vi "Load Products.vi"(8 "error in (no error)":errorcluster, 11 "Spanish Picker in":refnum<class "Spanish Picker.lvclass">) -> (0 "error out":errorcluster, 3 "Spanish Picker out":refnum<class "Spanish Picker.lvclass">)   [LabVIEW 2020, in "Spanish Picker.lvlib" / "Spanish Picker.lvclass"]
uses:
  Spanish Picker.lvclass
  D:/Storage/Source Code/Clase AF/ClaseAF/05 AF Camera/Products Picker/Products Picker.lvclass
  Products Picker/Products Picker.lvclass/Products Picker.ctl
  Products Picker/Products Picker.lvclass
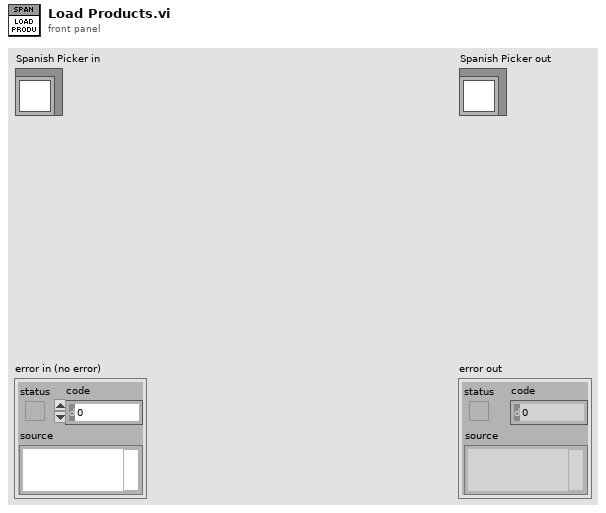
[diagram p1: front panel]
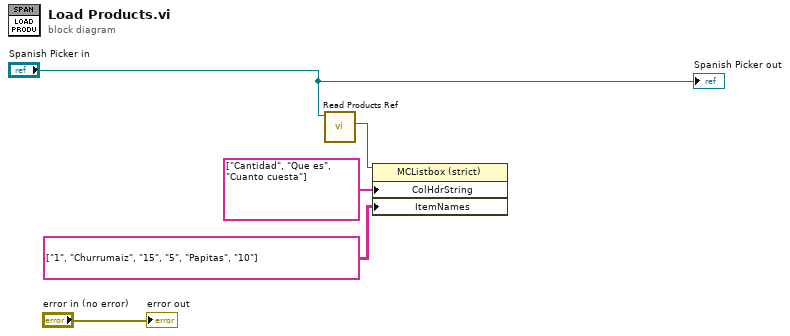
[diagram p0: block diagram]
diagram:
  n1 = call "Read Products Ref.vi"("Products Picker in"="Spanish Picker in") -> ("Products Ref"=w1:refnum<vi>)  [unwired: 9 in, 1 out]
  n2 = property class="MCListbox (strict)"(reference=w1, "ColHdrString"=string[] ["Cantidad", "Que es", "Cuanto cuesta"] ("Column Header Strings[]"), "ItemNames"=string[][] [["1", "Churrumaiz", "15"], ["5", "Papitas", "10"]] ("Item Names")) -> ()  [unwired: 1 in, 2 out]
  "error out" <- "error in (no error)"
  "Spanish Picker out" <- "Spanish Picker in"
